vi "Stop Point on Target.vi"(7 "Point Ident":string, 8 "error in":errorcluster, 11 "ISeries Actor in":refnum<class "ISeries Actor.lvclass">) -> (0 "error out":errorcluster, 3 "ISeries Actor out":refnum<class "ISeries Actor.lvclass">)   [LabVIEW 2023, in "ISeries Actor.lvlib" / "ISeries Actor.lvclass"]
uses:
  ISeries Actor.lvclass
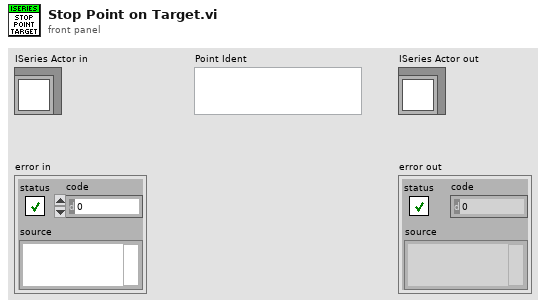
[diagram p1: front panel]
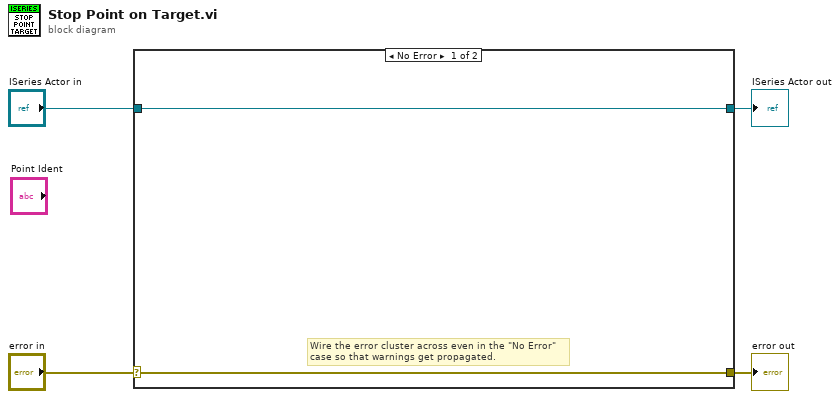
[diagram p0: block diagram]
diagram:
  n1 = case shown="No Error" "error in" {
    selector: "error in" -> [w5 w8]
    tunnel: [w5 w8] -> w3
    tunnel: [w6 w7] -> w1
    tunnel: "ISeries Actor in" -> [w6 w7]
    frame No Error {
      # "Wire the error cluster across even in the \"No Error\"\ncase so that warnings get propagated."
    }
    frame Error {
    }
  }
  "error out" <- w3
  "ISeries Actor out" <- w1
